vi "json_AddRightBrace.vi"(1 "ReadCMD_0":string="{\"ID\": \"b9b762fb-e465-4f6a-bde5-995dda67237b\", \"TO\": \"845CF3525B43\", \"FROM\": \"C87F542F1180\", \"CMD\": 0, \"CONTENT\": [{\"HOSTNAME\": \"SI-AGT01\", \"MAC\": \"845CF3525B43\", \"IP\": \"172.20.10.10\", \"CENTER_NAME\": \"C87F542F1180\", \"ADD_TOPIC\": \"topic/PC/845CF3525B43\", \"REQ_ID\": \"38A46EA6-1EA1-4C1D-82A7-A29BD9BCAD25\"}], \"STATUS\": true, \"ERRCODE\": \"\", \"ERRMSG\": \"\", \"TIMESTAMP\": 1759035794}") -> (0 "+}":string)   [LabVIEW 2020]
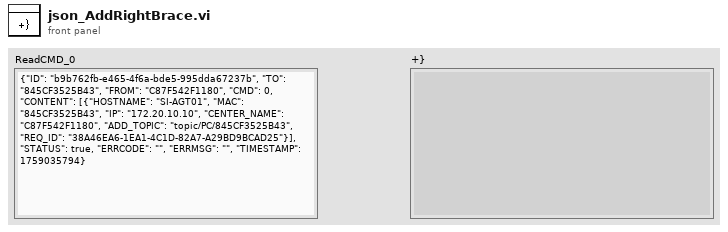
[diagram p1: front panel]
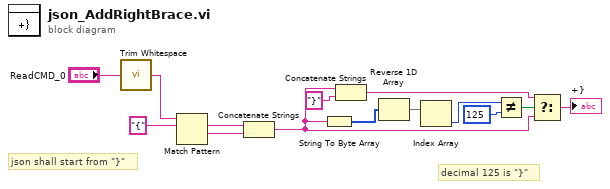
[diagram p0: block diagram]
diagram:
  # "json shall start from \"}\""
  # "decimal 125 is \"}\""
  n1 = call <vilib>:"Trim Whitespace.vi"("string"="ReadCMD_0") -> ("trimmed string"=w5:string)  [unwired: 1 in]
  n2 = Match Pattern(string=w5, regular expression="{") -> (match substring=w3:string, after substring=w2:string)  [unwired: 1 in, 2 out]
  n3 = Concatenate Strings(w3, w2) -> (w1:string)
  n4 = String To Byte Array(string=w1) -> (unsigned byte array=w14:u8[])
  n5 = Concatenate Strings(w1, "}" ("string")) -> (w8:string)
  n6 = Reverse 1D Array(array=w14) -> (reversed array=w13:u8[])
  n7 = Index Array(array=w13) -> (element=w12:u8)  [unwired: 1 in]
  n8 = Not Equal?(x=w12, y=u8 125 ("element")) -> (x != y?=w10:bool)
  n9 = Select(t=w8, s=w10, f=w1) -> (s? t:f=→"+}":string)
